vi "Calculate UE9 Stream Resolution.vi"(10 "Sample Rate":dbl format="%.2f") -> (2 "Resolution":i32=12)   [LabVIEW 2020]
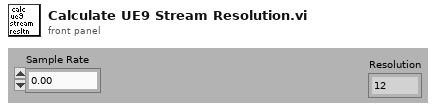
[diagram p1: front panel]
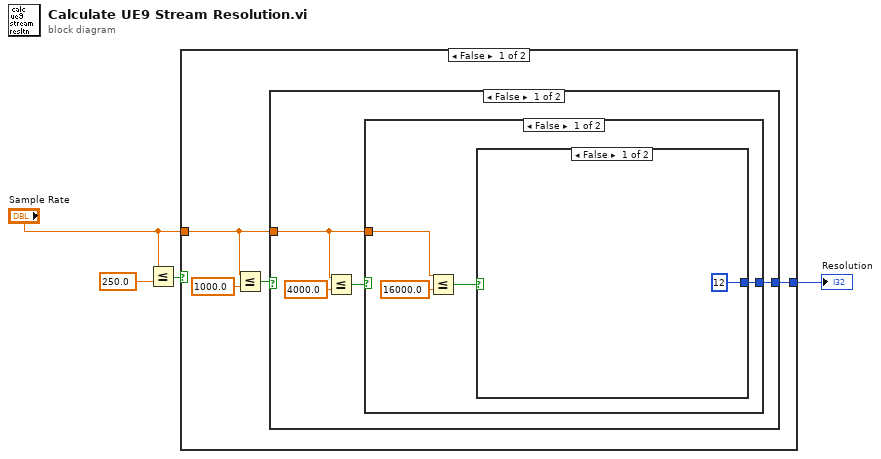
[diagram p0: block diagram]
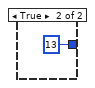
[diagram p2: hidden frame]
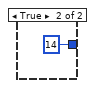
[diagram p3: hidden frame]
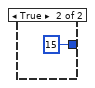
[diagram p4: hidden frame]
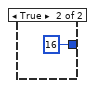
[diagram p5: hidden frame]
diagram:
  n1 = Less Or Equal?(x="Sample Rate", y=250.0) -> (x <= y?=w3:bool)
  n2 = case shown="False" w3 {
    tunnel: [w6 16] -> w2
    tunnel: "Sample Rate" -> [w5 _]
    frame False {
      n3 = Less Or Equal?(x=w5, y=1000.0) -> (x <= y?=w7:bool)
      n4 = case shown="False" w7 {
        tunnel: [w10 15] -> w6
        tunnel: w5 -> [w9 _]
        frame False {
          n5 = Less Or Equal?(x=w9, y=4000.0) -> (x <= y?=w11:bool)
          n6 = case shown="False" w11 {
            tunnel: [w14 14] -> w10
            tunnel: w9 -> [w13 _]
            frame False {
              n7 = Less Or Equal?(x=w13, y=16000.0) -> (x <= y?=w15:bool)
              n8 = case shown="False" w15 {
                tunnel: [12 13] -> w14
                frame False {
                }
                frame True {
                }
              }
            }
            frame True {
            }
          }
        }
        frame True {
        }
      }
    }
    frame True {
    }
  }
  "Resolution" <- w2
